vi "Init.vi"(8 "error in (no error)":errorcluster, 11 "Path":path) -> (0 "error out":errorcluster)   [LabVIEW 2020, in "Logger.lvlib"]
uses:
  Logger.lvlib
  LoggerGlobal.vi
  Event.ctl
panel:
  in  "Event":T1
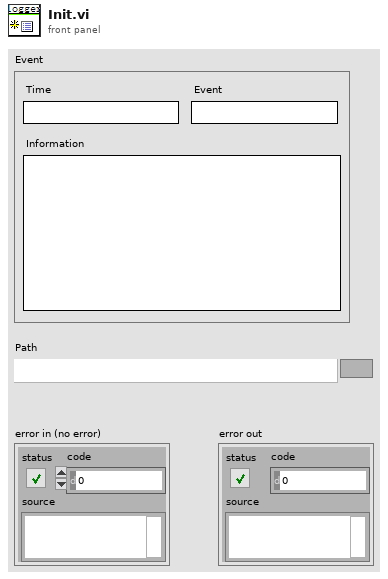
[diagram p1: front panel]
types:
  T1 = typedef "Logger.lvlib/Event.ctl" = cluster{"Time":string, "Event":string, "Information":string}
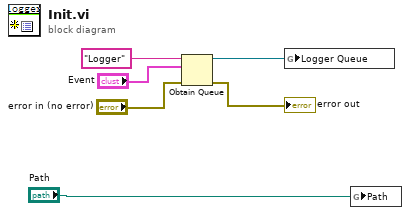
[diagram p0: block diagram]
diagram:
  n1 = Obtain Queue(name (unnamed)="Logger", element data type="Event", error in (no error)="error in (no error)") -> (queue out=w1:refnum<queue>, error out=→"error out":errorcluster)  [unwired: 2 in, 1 out]
  n2 = global write "LoggerGlobal.vi" "Logger Queue"(w1) -> ()
  n3 = global write "LoggerGlobal.vi" "Path"("Path") -> ()
